vi "Histogram.vi"(5 "Current Block No":i32=1, 6 "No of bins":i32, 7 "Shift Hist":i32[](array[numeric]), 8 "Min value":dbl format="%.2f", 9 "Max value":dbl format="%.2f", 10 "X":dbl[](array[numeric]) format="%.2f") -> (0 "Shift Hist":i32[](array[numeric]), 1 "Histogram of X":dbl[](array[numeric]) format="%.4f", 3 "Axis":dbl[](array[numeric]) format="%.2f")   [LabVIEW 2010]
uses:
  <vilib>/Analysis/NI_AALPro.lvlib
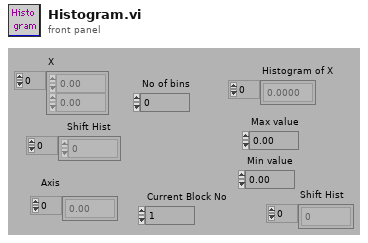
[diagram p1: front panel]
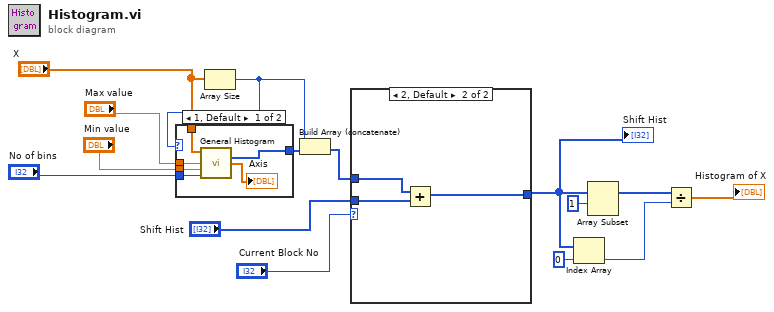
[diagram p0: block diagram]
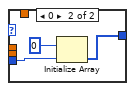
[diagram p2: hidden frame]
diagram:
  n1 = Array Size(array="X") -> (size(s)=w2:i32)
  n2 = case shown="1, Default" w2 {
    tunnel: "Max value" -> [w21 _]
    tunnel: "Min value" -> [w20 _]
    tunnel: [w18 w22] -> w11
    tunnel: "X" -> [w17 _]
    tunnel: "No of bins" -> [w19 w24]
    frame 1, Default {
      n3 = call <vilib>:"General Histogram.vi"("X"=w17, "max"=w21, "min"=w20, "# bins"=w19) -> ("Histogram"=w18:i32[], "Axis"=→"Axis":dbl[])  [unwired: 2 in, 8 out]
    }
    frame 0 {
      n4 = Initialize Array(0 ("Element Data"), w24) -> (w22:i32[])
    }
  }
  n5 = Build Array (concatenate)(w2, w11) -> (w9:i32[])
  n6 = case shown="2, Default" "Current Block No" {
    tunnel: [w25 w28] -> w4
    tunnel: w9 -> [w25 w27]
    tunnel: "Shift Hist" -> [_ w26]
    frame 1 {
    }
    frame 2, Default {
      n7 = Add(x=w27, y=w26) -> (x+y=w28:i32[])
    }
  }
  "Shift Hist" <- w4
  n8 = Index Array(array=w4, index=0 ("Index")) -> (element=w3:i32)
  n9 = Array Subset(array=w4, index=1 ("Array Index")) -> (w7:i32[])  [unwired: 1 in]
  n10 = Divide(x=w7, y=w3) -> (x/y=→"Histogram of X":dbl[])
